vi "flash.vi"(0 "Boolean 2":bool) -> (8 "Numeric":dbl)   [LabVIEW 2019]
panel:
  out "Boolean 3":bool
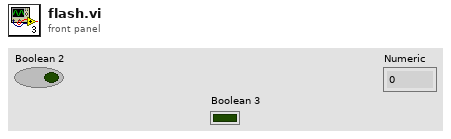
[diagram p1: front panel]
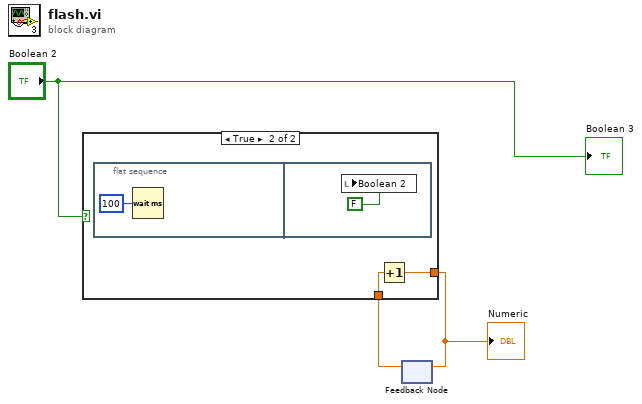
[diagram p0: block diagram]
diagram:
  n1 = feedback #1() -> (w2:dbl)  [unwired: 1 in]
  n2 = case shown="True" "Boolean 2" {
    tunnel: [w4 w6] -> w1
    tunnel: w2 -> [w4 w5]
    frame False {
    }
    frame True {
      n3 = flat-sequence {
        frame #0 {
          n4 = Wait (ms)(milliseconds to wait=u32 100) -> ()  [unwired: 1 out]
        }
        frame #1 {
          n5 = local write "Boolean 2"(FALSE) -> ()
        }
      }
      n6 = Increment(x=w5) -> (x+1=w6:dbl)
    }
  }
  "Numeric" <- w1
  n7 = feedback-in #1(w1) -> ()
  "Boolean 3" <- "Boolean 2"
